vi "CalculateServoAngle.vi"() -> ()   [LabVIEW 2012]
panel:
  out "Output Pulsewidth (uSec)":i32
  in  "Input angle (rad)":dbl
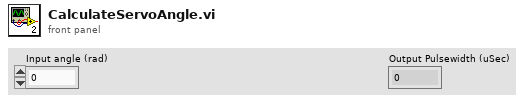
[diagram p1: front panel]
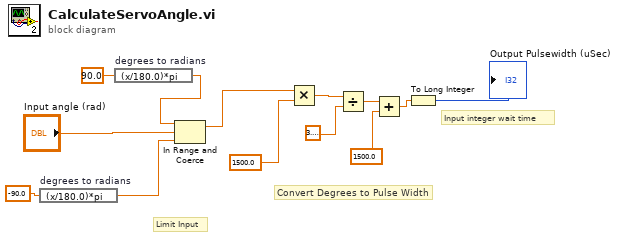
[diagram p0: block diagram]
diagram:
  # "Input integer wait time"
  # "Convert Degrees to Pulse Width"
  # "Limit Input"
  n1 = expression code="(x/180.0)*pi" "degrees to radians"(-90.0 ("lower limit")) -> (w4:dbl)
  n2 = expression code="(x/180.0)*pi" "degrees to radians"(90.0 ("upper limit")) -> (w3:dbl)
  n3 = In Range and Coerce(upper limit=w3, x="Input angle (rad)", lower limit=w4) -> (coerced(x)=w13:dbl)  [unwired: 1 out]
  n4 = Multiply(x=w13, y=1500.0) -> (x*y=w12:dbl)
  n5 = Divide(x=w12, y=3.141592653589793) -> (x/y=w10:dbl)
  n6 = Add(x=w10, y=1500.0) -> (x+y=w9:dbl)
  n7 = To Long Integer(number=w9) -> (32bit integer=→"Output Pulsewidth (uSec)":i32)
